vi "Stop Command.vi"(8 "error in (no error)":errorcluster, 10 "Is Command Finished?":bool, 11 "System Actor in":refnum<class "System Actor.lvclass">) -> (0 "error out":errorcluster, 3 "System Actor out":refnum<class "System Actor.lvclass">)   [LabVIEW 2013, in "Robot Actors.lvlib" / "System Actor.lvlib" / "System Actor.lvclass"]
uses:
  System Actor.lvclass
  <vilib>/ActorFramework/Message Enqueuer/Message Enqueuer.lvclass
  System Actor.lvclass/System Actor.ctl
  <vilib>/ActorFramework/Stop Msg/Stop Msg.lvclass/Stop Msg.ctl
  <vilib>/ActorFramework/Message Enqueuer/Message Enqueuer.lvclass/Message Enqueuer.ctl
  <vilib>/ActorFramework/Message Enqueuer/Enqueue Critical.vi
  <vilib>/ActorFramework/Message Enqueuer/Enqueue.vi
  <vilib>/ActorFramework/Message Priority Queue/Priority Enqueue.vi
  <vilib>/ActorFramework/Stop Msg/Stop Msg.lvclass
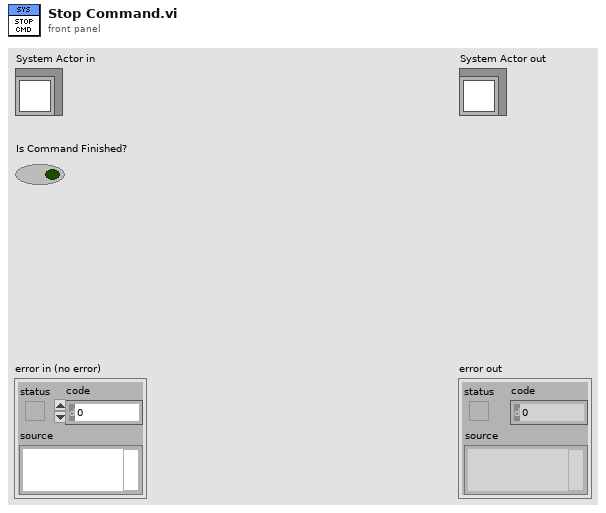
[diagram p1: front panel]
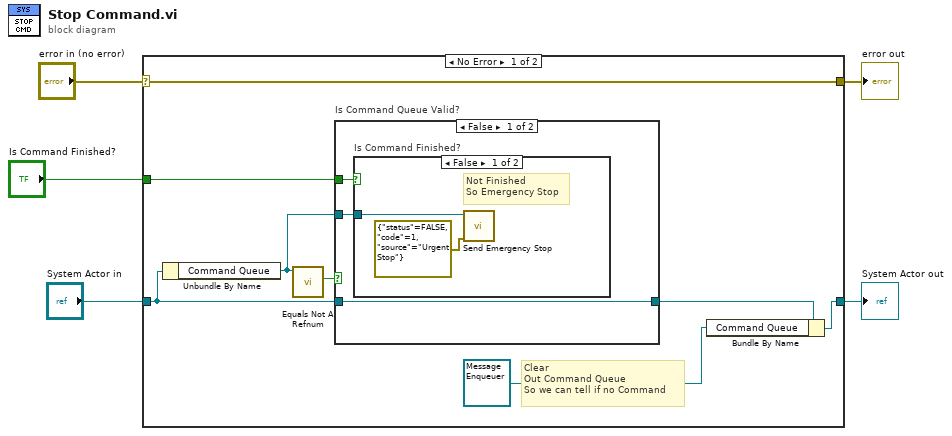
[diagram p0: block diagram]
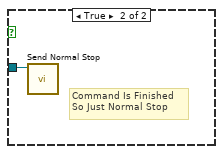
[diagram p2: hidden frame]
diagram:
  n1 = case shown="No Error" "error in (no error)" {
    selector: "error in (no error)" -> [w13 w22]
    tunnel: [w13 w22] -> w4
    tunnel: [w12 w21] -> w2
    tunnel: "System Actor in" -> [w6 w21]
    tunnel: "Is Command Finished?" -> [w7 _]
    frame No Error {
      # "Clear\nOut Command Queue\nSo we can tell if no Command"
      n2 = Unbundle By Name(w6) -> ("Command Queue"=w10:refnum<class "Message Enqueuer.lvclass">)
      n3 = call <vilib>:"Equals Not A Refnum.vi"("Message Enqueuer"=w10) -> ("Not a refnum?"=w9:bool)  [unwired: 10 in]
      n4 = case "Is Command Queue Valid?" shown="False" w9 {
        tunnel: w10 -> [w16 _]
        tunnel: [w14 w20] -> w8
        tunnel: w7 -> [w15 _]
        tunnel: w6 -> [w14 w20]
        frame False {
          n5 = case "Is Command Finished?" shown="False" w15 {
            tunnel: w16 -> [w18 w19]
            frame False {
              # "Not Finished\nSo Emergency Stop"
              n6 = call <vilib>:"Send Emergency Stop.vi"("error in (no error)"=errorcluster {"status"=FALSE, "code"=1, "source"="Urgent Stop"}, "Message Enqueuer"=w18) -> ()  [unwired: 9 in, 1 out]
            }
            frame True {
              # "Command Is Finished\nSo Just Normal Stop"
              n7 = call <vilib>:"Send Normal Stop.vi"("Message Enqueuer"=w19) -> ()  [unwired: 10 in, 1 out]
            }
          }
        }
        frame True {
          # "Command Queue Is\nNot Valid so No Command\nTo Stop"
        }
      }
      n8 = Bundle By Name(cluster=w8, "Command Queue"=refnum<class "Message Enqueuer.lvclass"> refnum) -> (w12:refnum<class "System Actor.lvclass">)
    }
    frame Error {
    }
  }
  "error out" <- w4
  "System Actor out" <- w2
